vi "Vision Processing.vi"(4 "error in (no error)":errorcluster, 7 "Image Size":T1=enum."320x240") -> ()   [LabVIEW 2017]
doc: "This VI runs in parallel to other tasks. It gets images from the camera, processes them for color or shape and use that information to affect robot behavior."
uses:
  <vilib>/Rock Robotics/WPI/Camera/WPI_CameraImageSize.ctl
  <vilib>/Rock Robotics/WPI/Camera/WPI_CameraWhite Balance Values.ctl
  <vilib>/Rock Robotics/WPI/Camera/WPI_CameraExposure Values.ctl
  <vilib>/Rock Robotics/WPI/Camera/WPI_CameraFrameRate.ctl
  Robot Global Data.vi
panel:
  in  "Image Size 2":T1=enum."320x240"
  in  "error in (no error) 2":errorcluster
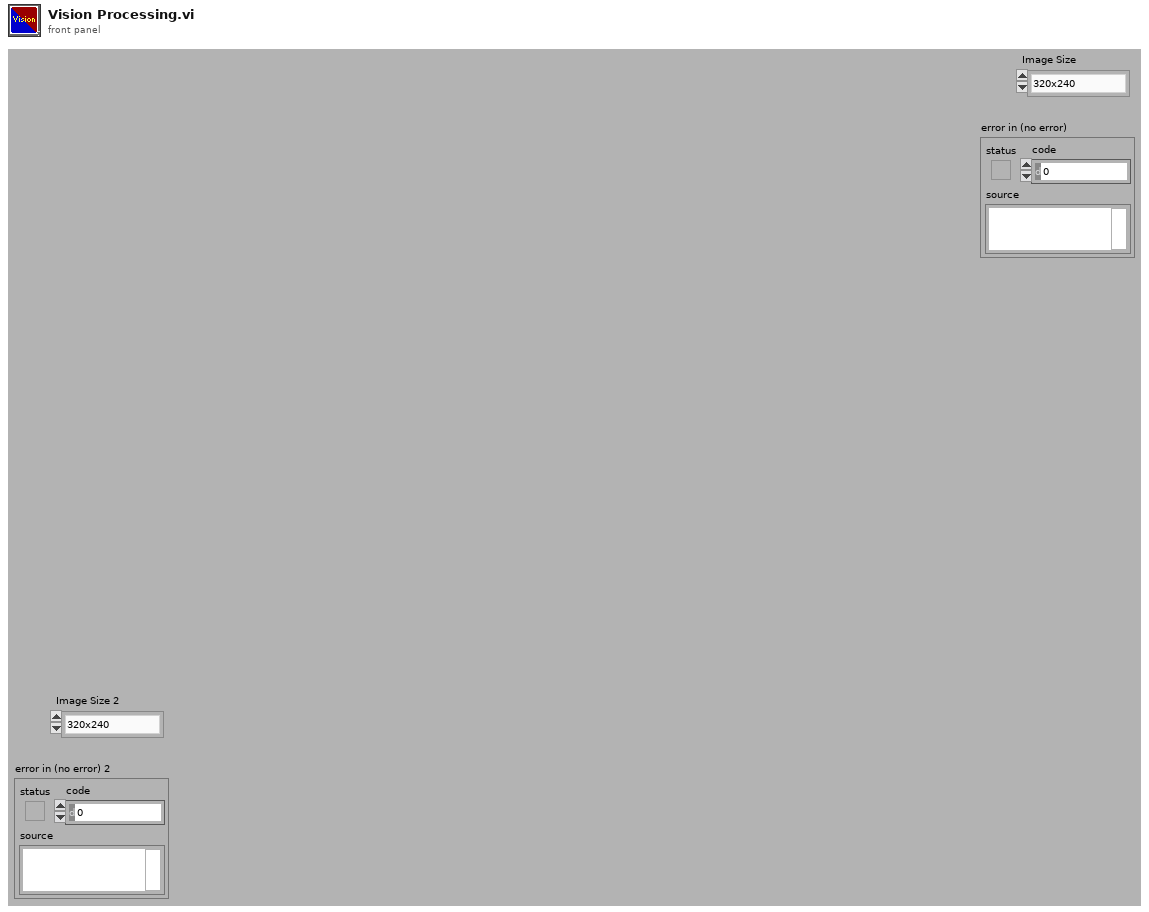
[diagram p1: front panel]
types:
  T1 = typedef "WPI_CameraImageSize.ctl" = enum16{"640x480", "320x240", "160x120", "Custom"}
  T2 = typedef "WPI_CameraFrameRate.ctl" = u32
  T3 = typedef "WPI_CameraExposure Values.ctl" = enum16{"Auto", "Flicker-free 50 Hz", "Flicker-free 60 Hz", "Hold current", "Custom"}
  T4 = typedef "WPI_CameraWhite Balance Values.ctl" = enum16{"Auto", "Fixed indoor", "Fixed outdoor 1", "Fixed outdoor 2", "Fixed fluorescent 1", "Fixed fluorescent 2", "Hold current", "Custom"}
  T5 = typedef "Image Type" = u32
  T6 = typedef "WPI_CameraDevRef.ctl" = cluster{"Camera Address":string, "CameraStatus":errorcluster}
  T7 = typedef "IMAQ Image.ctl" = refnum<image>
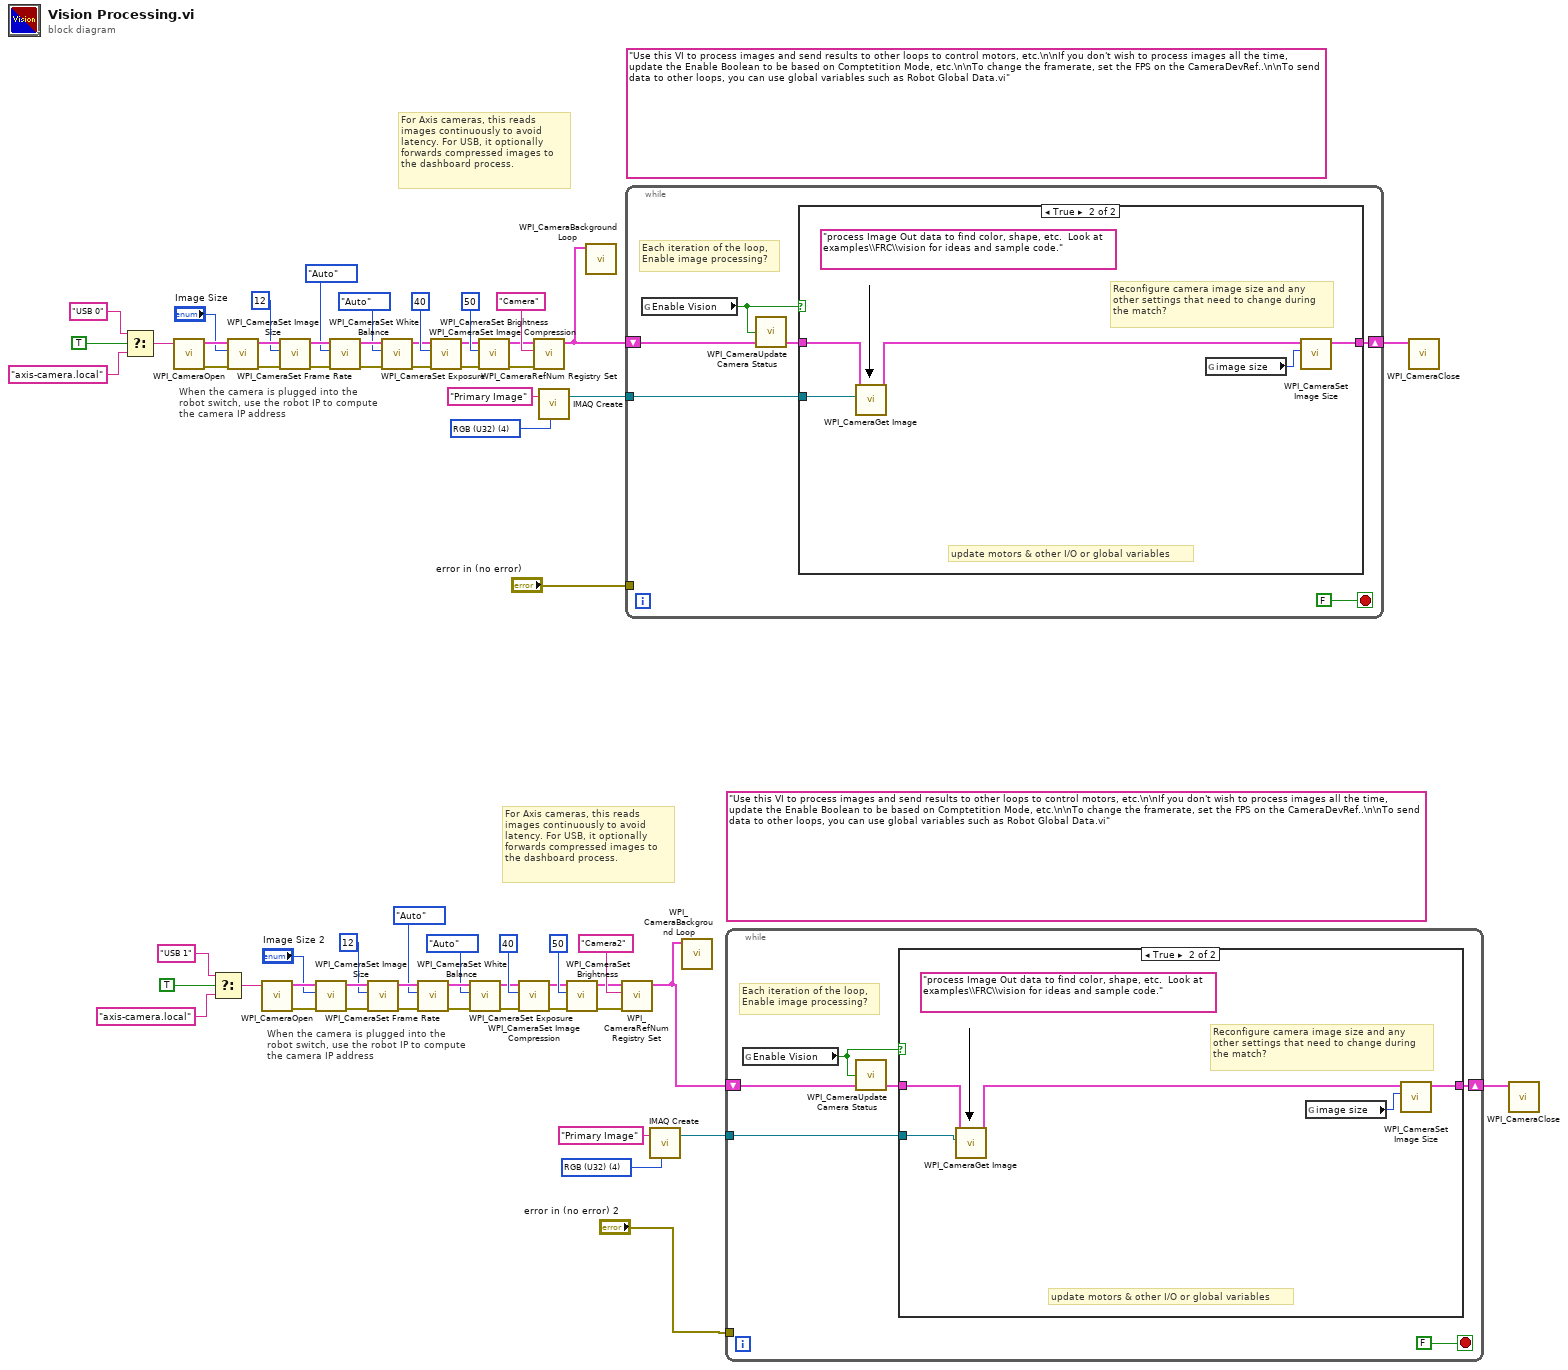
[diagram p0: block diagram]
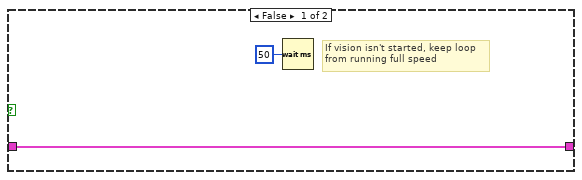
[diagram p2: hidden frame]
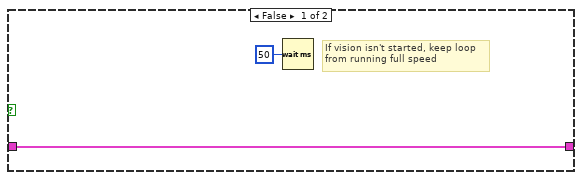
[diagram p3: hidden frame]
diagram:
  (unwired) "Use this VI to process images and send results to other loops to control motors, etc.\n\nIf you don't wish to process images all the time, update the Enable Boolean to be based on Comptetition Mode, etc.\n\nTo change the framerate, set the FPS on the CameraDevRef..\n\nTo send data to other loops, you can use global variables such as Robot Global Data.vi"
  w31 = T5 4 items=["Grayscale (U8)", "Grayscale (I16)", "Grayscale (SGL)", "Complex (CSG)", "RGB (U32)", "HSL (U32)", "RGB (U64)"] ("Image Type")
  (unwired) "Use this VI to process images and send results to other loops to control motors, etc.\n\nIf you don't wish to process images all the time, update the Enable Boolean to be based on Comptetition Mode, etc.\n\nTo change the framerate, set the FPS on the CameraDevRef..\n\nTo send data to other loops, you can use global variables such as Robot Global Data.vi"
  w62 = T5 4 items=["Grayscale (U8)", "Grayscale (I16)", "Grayscale (SGL)", "Complex (CSG)", "RGB (U32)", "HSL (U32)", "RGB (U64)"] ("Image Type")
  # "For Axis cameras, this reads\nimages continuously to avoid\nlatency. For USB, it optionally\nforwards compressed images to\nthe dashboard process."
  # "When the camera is plugged into the\nrobot switch, use the robot IP to compute\nthe camera IP address"
  # "When the camera is plugged into the\nrobot switch, use the robot IP to compute\nthe camera IP address"
  # "For Axis cameras, this reads\nimages continuously to avoid\nlatency. For USB, it optionally\nforwards compressed images to\nthe dashboard process."
  n1 = Select(t="USB 0" ("format string"), s=TRUE ("dot notation? (F)"), f="axis-camera.local" ("format string")) -> (s? t:f=w33:string)
  n2 = call <vilib>:"WPI_CameraOpen.vi"("Camera Address"=w33) -> ("error out"=w50:errorcluster, "CameraDevRef"=w51:T6)  [unwired: 1 in, 8 out]
  n3 = Select(t="USB 1" ("format string"), s=TRUE ("dot notation? (F)"), f="axis-camera.local" ("format string")) -> (s? t:f=w6:string)
  n4 = call <vilib>:"WPI_CameraSet Image Size.vi"("error in (no error)"=w50, "Image Size"="Image Size", "CameraDevRef"=w51) -> ("error out"=w49:errorcluster, "CameraDevRef Out"=w52:T6)  [unwired: 1 in, 6 out]
  n5 = call <vilib>:"WPI_CameraOpen.vi"("Camera Address"=w6) -> ("error out"=w20:errorcluster, "CameraDevRef"=w21:T6)  [unwired: 1 in, 8 out]
  n6 = call <vilib>:"WPI_CameraSet Frame Rate.vi"("error in (no error)"=w49, "Frame Rate (fps)"=T2 12, "CameraDevRef"=w52) -> ("error out"=w48:errorcluster, "CameraDevRef Out"=w54:T6)  [unwired: 7 out]
  n7 = call <vilib>:"WPI_CameraSet Image Size.vi"("error in (no error)"=w20, "Image Size"="Image Size 2", "CameraDevRef"=w21) -> ("error out"=w19:errorcluster, "CameraDevRef Out"=w22:T6)  [unwired: 1 in, 6 out]
  n8 = call <vilib>:"WPI_CameraSet White Balance.vi"("error in (no error)"=w48, "White Balance"=WPI_CameraWhite_Balance_Values."Auto", "CameraDevRef"=w54) -> ("error out"=w47:errorcluster, "CameraDevRef Out"=w53:T6)  [unwired: 1 in, 6 out]
  n9 = call <vilib>:"WPI_CameraSet Frame Rate.vi"("error in (no error)"=w19, "Frame Rate (fps)"=T2 12, "CameraDevRef"=w22) -> ("error out"=w18:errorcluster, "CameraDevRef Out"=w24:T6)  [unwired: 7 out]
  n10 = call <vilib>:"WPI_CameraSet Exposure.vi"("error in (no error)"=w47, "Exposure"=WPI_CameraExposure_Values."Auto", "CameraDevRef"=w53) -> ("error out"=w46:errorcluster, "CameraDevRef Out"=w56:T6)  [unwired: 1 in, 6 out]
  n11 = call <vilib>:"WPI_CameraSet White Balance.vi"("error in (no error)"=w18, "White Balance"=WPI_CameraWhite_Balance_Values."Auto", "CameraDevRef"=w24) -> ("error out"=w17:errorcluster, "CameraDevRef Out"=w23:T6)  [unwired: 1 in, 6 out]
  n12 = call <vilib>:"WPI_CameraSet Image Compression.vi"("error in (no error)"=w46, "Compression"=40, "CameraDevRef"=w56) -> ("error out"=w45:errorcluster, "CameraDevRef Out"=w55:T6)  [unwired: 7 out]
  n13 = call <vilib>:"WPI_CameraSet Exposure.vi"("error in (no error)"=w17, "Exposure"=WPI_CameraExposure_Values."Auto", "CameraDevRef"=w23) -> ("error out"=w16:errorcluster, "CameraDevRef Out"=w26:T6)  [unwired: 1 in, 6 out]
  n14 = call <vilib>:"WPI_CameraSet Brightness.vi"("error in (no error)"=w45, "Brightness"=50, "CameraDevRef"=w55) -> ("error out"=w43:errorcluster, "CameraDevRef Out"=w44:T6)  [unwired: 1 in, 6 out]
  n15 = call <vilib>:"WPI_CameraSet Image Compression.vi"("error in (no error)"=w16, "Compression"=40, "CameraDevRef"=w26) -> ("error out"=w15:errorcluster, "CameraDevRef Out"=w25:T6)  [unwired: 7 out]
  n16 = call <vilib>:"WPI_CameraRefNum Registry Set.vi"("error in (no error)"=w43, "refnum name"="Camera", "CameraDevRef"=w44) -> ("CameraDevRef"=w39:T6)  [unwired: 1 in, 7 out]
  n17 = call "IMAQ Create"("Image Name"="Primary Image", "Image Type"=w62) -> ("New Image"=w60:T7)  [unwired: 2 in, 2 out]
  n18 = call <vilib>:"WPI_CameraSet Brightness.vi"("error in (no error)"=w15, "Brightness"=50, "CameraDevRef"=w25) -> ("error out"=w13:errorcluster, "CameraDevRef Out"=w14:T6)  [unwired: 1 in, 6 out]
  n19 = call <vilib>:"WPI_CameraBackground Loop.vi"("CameraDevRef"=w39) -> ()  [unwired: 11 in]
  n20 = call <vilib>:"WPI_CameraRefNum Registry Set.vi"("error in (no error)"=w13, "refnum name"="Camera2", "CameraDevRef"=w14) -> ("CameraDevRef"=w2:T6)  [unwired: 1 in, 7 out]
  n21 = while {
    shift-right: [w67] -> w37
    shift-left: w39 -> [w65]
    tunnel: w60 -> [w66]
    tunnel: "error in (no error)" -> [_]
    stop <- FALSE stop-if-true
    # "Each iteration of the loop,\nEnable image processing?"
    n22 = global read "Robot Global Data.vi" "Enable Vision"() -> (w63:bool)
    n23 = call <vilib>:"WPI_CameraUpdate Camera Status.vi"("CameraDevRef In"=w65, "Enable Vision"=w63) -> ("CameraDevRef Out"=w64:T6)  [unwired: 3 in]
    n24 = case shown="True" w63 {
      tunnel: w66 -> [_ w74]
      tunnel: [w70 w75] -> w67
      tunnel: w64 -> [w70 w72]
      frame False {
        # "If vision isn't started, keep loop\nfrom running full speed"
        n25 = Wait (ms)(milliseconds to wait=u32 50) -> ()  [unwired: 1 out]
      }
      frame True {
        (unwired) "process Image Out data to find color, shape, etc.  Look at examples\\FRC\\vision for ideas and sample code."
        # "update motors & other I/O or global variables"
        # "Reconfigure camera image size and any\nother settings that need to change during\nthe match?"
        n26 = call <vilib>:"WPI_CameraGet Image.vi"("Image"=w74, "CameraDevRef"=w72) -> ("CameraDevRef Out"=w71:T6)  [unwired: 1 in, 8 out]
        n27 = global read "Robot Global Data.vi" "image size"() -> (w73:T1)
        n28 = call <vilib>:"WPI_CameraSet Image Size.vi"("Image Size"=w73, "CameraDevRef"=w71) -> ("CameraDevRef Out"=w75:T6)  [unwired: 2 in, 7 out]
      }
    }
  }
  n29 = call "IMAQ Create"("Image Name"="Primary Image", "Image Type"=w31) -> ("New Image"=w1:T7)  [unwired: 2 in, 2 out]
  n30 = call <vilib>:"WPI_CameraBackground Loop.vi"("CameraDevRef"=w2) -> ()  [unwired: 11 in]
  n31 = while {
    shift-right: [w80] -> w4
    shift-left: w2 -> [w79]
    tunnel: "error in (no error) 2" -> [_]
    tunnel: w1 -> [w76]
    stop <- FALSE stop-if-true
    # "Each iteration of the loop,\nEnable image processing?"
    n32 = global read "Robot Global Data.vi" "Enable Vision"() -> (w77:bool)
    n33 = call <vilib>:"WPI_CameraUpdate Camera Status.vi"("CameraDevRef In"=w79, "Enable Vision"=w77) -> ("CameraDevRef Out"=w78:T6)  [unwired: 3 in]
    n34 = case shown="True" w77 {
      tunnel: [w83 w88] -> w80
      tunnel: w78 -> [w83 w86]
      tunnel: w76 -> [_ w84]
      frame False {
        # "If vision isn't started, keep loop\nfrom running full speed"
        n35 = Wait (ms)(milliseconds to wait=u32 50) -> ()  [unwired: 1 out]
      }
      frame True {
        (unwired) "process Image Out data to find color, shape, etc.  Look at examples\\FRC\\vision for ideas and sample code."
        # "update motors & other I/O or global variables"
        # "Reconfigure camera image size and any\nother settings that need to change during\nthe match?"
        n36 = call <vilib>:"WPI_CameraGet Image.vi"("Image"=w84, "CameraDevRef"=w86) -> ("CameraDevRef Out"=w85:T6)  [unwired: 1 in, 8 out]
        n37 = global read "Robot Global Data.vi" "image size"() -> (w87:T1)
        n38 = call <vilib>:"WPI_CameraSet Image Size.vi"("Image Size"=w87, "CameraDevRef"=w85) -> ("CameraDevRef Out"=w88:T6)  [unwired: 2 in, 7 out]
      }
    }
  }
  n39 = call <vilib>:"WPI_CameraClose.vi"("CameraDevRef"=w37) -> ()  [unwired: 1 in, 10 out]
  n40 = call <vilib>:"WPI_CameraClose.vi"("CameraDevRef"=w4) -> ()  [unwired: 1 in, 10 out]
